vi "GetHelp.vi"(0 "XRef":T20, 1 "Point":T19, 2 "State In":T14) -> (14 "Standard Help Info":T12, 15 "Detailed Help Info":T9, 16 "Subitem Help Info":T3, 17 "Use Detailed Help?":T2, 18 "Use Subitem Help?":T2, 19 "Fatal Error Out":T1)   [LabVIEW 2021, in "myRIO AudioOut N Samples Open.xnode"]
doc: "Opens a reference to one or more audio output channels, which you use to perform n samples write operations. You must open a reference before you write values to an audio output channel."
uses:
  <vilib>/myRIO/Instrument Drivers/Onboard IO/AudioOut Block/vis/myRIO AudioOut N Samples Open.xnode
  <vilib>/XNodeSupport/XNodeXNodeRef.ctl
  <vilib>/XNodeSupport/XNodePoint.ctl
  <vilib>/XNodeSupport/XNodeInt.ctl
  <vilib>/myRIO/Instrument Drivers/Onboard IO/AudioOut Block/vis/State.ctl
  <vilib>/myRIO/Common/Instrument Driver Framework/Utilities/typedefs/myRIOXPeripheral.ctl
  <vilib>/XNodeSupport/XNodeTerm4Array.ctl
  <vilib>/XNodeSupport/XNodeTerm4.ctl
  <vilib>/XNodeSupport/XNodeString.ctl
  <vilib>/XNodeSupport/XNodeVariant.ctl
  <vilib>/XNodeSupport/XNodeRect32.ctl
  <vilib>/XNodeSupport/XNodeBool.ctl
  <vilib>/XNodeSupport/XNodeTermDirection.ctl
  <vilib>/XNodeSupport/XNodeStandardHelpInfo.ctl
  <vilib>/XNodeSupport/XNodePath.ctl
  <vilib>/XNodeSupport/XNodeDetailedHelpInfo.ctl
  <vilib>/XNodeSupport/XNodeImage.ctl
  <vilib>/XNodeSupport/XNodeTerms.ctl
  <vilib>/XNodeSupport/XNodeTerm.ctl
  <vilib>/XNodeSupport/XNodeSubitemHelpInfo.ctl
  <vilib>/XNodeSupport/XNodeErrorCluster.ctl
  <vilib>/myRIO/Common/Instrument Driver Framework/Utilities/vis/myRIOXGlobal.vi
  <vilib>/XNodeSupport/NI_XNodeSupport.lvlib
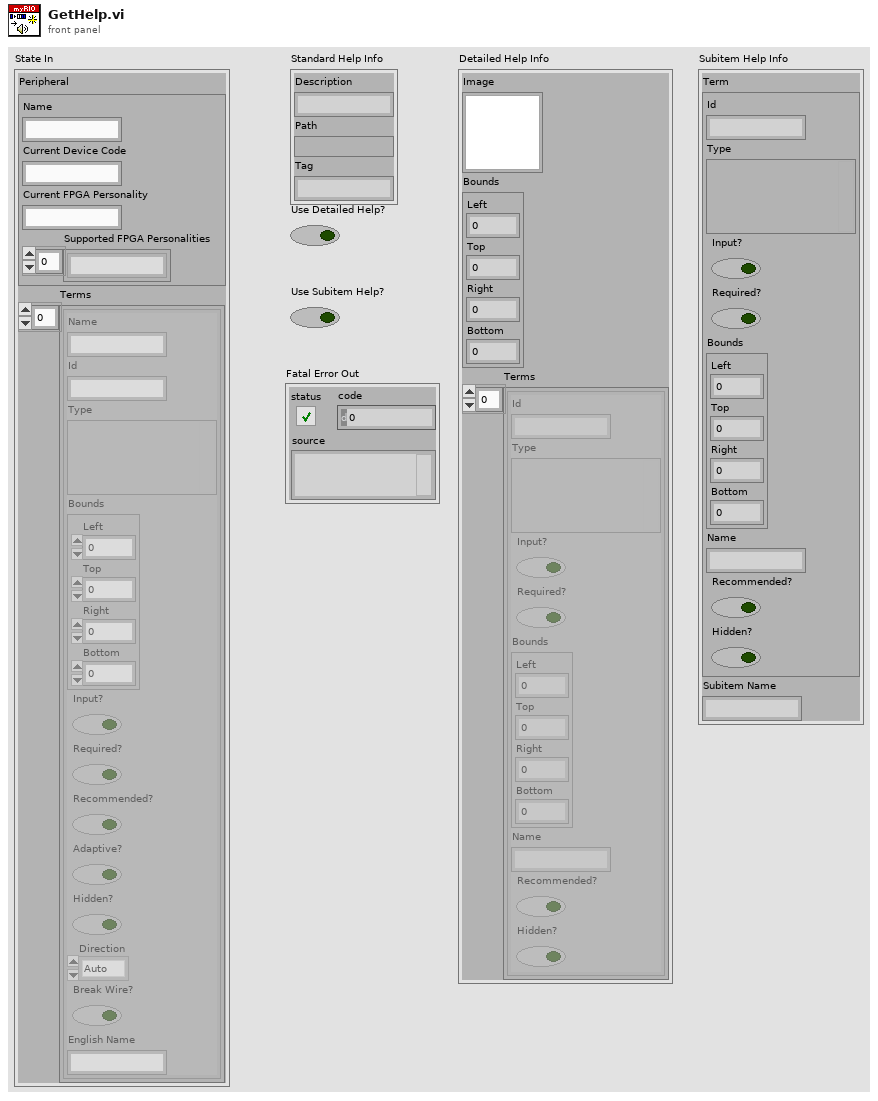
[diagram p1: front panel]
types:
  T1 = typedef "NI_XNodeSupport.lvlib/XNodeErrorCluster.ctl" = errorcluster
  T2 = typedef "NI_XNodeSupport.lvlib/XNodeBool.ctl" = bool
  T3 = typedef "NI_XNodeSupport.lvlib/XNodeSubitemHelpInfo.ctl" = cluster{"Term":T4, "Subitem Name":T5}
  T4 = typedef "NI_XNodeSupport.lvlib/XNodeTerm.ctl" = cluster{"Id":T5, "Type":T6, "Input?":T2, "Required?":T2, "Bounds":T7, "Name":T5, "Recommended?":T2, "Hidden?":T2}
  T5 = typedef "NI_XNodeSupport.lvlib/XNodeString.ctl" = string
  T6 = typedef "NI_XNodeSupport.lvlib/XNodeVariant.ctl" = variant
  T7 = typedef "NI_XNodeSupport.lvlib/XNodeRect32.ctl" = cluster{"Left":T8, "Top":T8, "Right":T8, "Bottom":T8}
  T8 = typedef "NI_XNodeSupport.lvlib/XNodeInt.ctl" = i32
  T9 = typedef "NI_XNodeSupport.lvlib/XNodeDetailedHelpInfo.ctl" = cluster{"Image":T10, "Bounds":T7, "Terms":T11}
  T10 = typedef "NI_XNodeSupport.lvlib/XNodeImage.ctl" = picture
  T11 = typedef "NI_XNodeSupport.lvlib/XNodeTerms.ctl" = T4[]
  T12 = typedef "NI_XNodeSupport.lvlib/XNodeStandardHelpInfo.ctl" = cluster{"Description":T5, "Path":T13, "Tag":T5}
  T13 = typedef "NI_XNodeSupport.lvlib/XNodePath.ctl" = path
  T14 = typedef "myRIO AudioOut N Samples Open.xnode/State.ctl" = cluster{"Peripheral":T15, "Terms":T16}
  T15 = typedef "myRIOXPeripheral.ctl" = cluster{"Name":string, "Current Device Code":string, "Current FPGA Personality":string, "Supported FPGA Personalities":string[]}
  T16 = typedef "NI_XNodeSupport.lvlib/XNodeTerm4Array.ctl" = T17[]
  T17 = typedef "NI_XNodeSupport.lvlib/XNodeTerm4.ctl" = cluster{"Name":T5, "Id":T5, "Type":T6, "Bounds":T7, "Input?":T2, "Required?":T2, "Recommended?":T2, "Adaptive?":T2, "Hidden?":T2, "Direction":T18, "Break Wire?":T2, "English Name":T5}
  T18 = typedef "NI_XNodeSupport.lvlib/XNodeTermDirection.ctl" = enum32{"Auto", "Up", "Down", "Left", "Right", "Center"}
  T19 = typedef "NI_XNodeSupport.lvlib/XNodePoint.ctl" = cluster{"H":T8, "V":T8}
  T20 = typedef "NI_XNodeSupport.lvlib/XNodeXNodeRef.ctl" = refnum<vi>
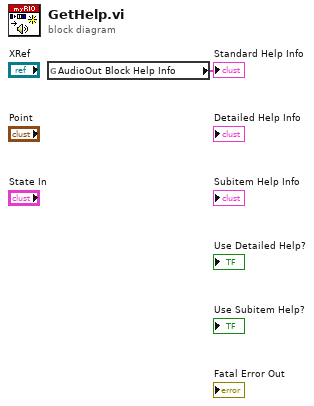
[diagram p0: block diagram]
diagram:
  n1 = global read "myRIOXGlobal.vi" "AudioOut Block Help Info"() -> (→"Standard Help Info":T12)
